vi "Fetch.vi"(8 "error in (no error)":errorcluster, 10 "Message in":refnum<class "FetchMessage.lvclass">, 11 "ExampleClassDScaffold in":refnum<class "ExampleClassDScaffold.lvclass">) -> (0 "error out":errorcluster, 3 "ExampleClassDScaffold out":refnum<class "ExampleClassDScaffold.lvclass">)   [LabVIEW 2012, in "ExampleClassDScaffold.lvclass"]
doc: "The fetch method processes the command 'fetch'.\n\nThe command 'fetch' is used for receiving various forms of data."
uses:
  ExampleClassDScaffold.lvclass
  <vilib>/Distrio/Murmex/FetchMessage/FetchMessage.lvclass
  <vilib>/Distrio/Murmex/Murmex/Murmex.lvclass
  <vilib>/Distrio/Murmex/Murmex/observer_cluster_2.ctl
  <vilib>/Distrio/Murmex/Murmex/observe_mode_enum.ctl
  <vilib>/Distrio/Murmex/Murmex/Queue type enum.ctl
  <vilib>/Distrio/Murmex/ProceedMessage/ProceedMessage.lvclass
  <vilib>/Distrio/Murmex/Message/Message.lvclass
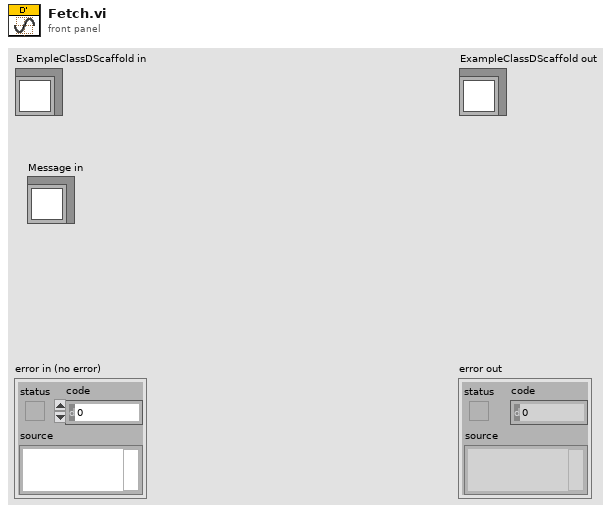
[diagram p1: front panel]
types:
  T1 = typedef "Murmex.lvlib/Murmex.lvclass/Queue type enum.ctl" = enum16{"RabbitMQ", "Network streaming queue"}
  T2 = typedef "Murmex.lvlib/Murmex.lvclass/observe_mode_enum.ctl" = enum16{"all data blocks", "only finished data blocks"}
  T3 = typedef "Murmex.lvlib/Murmex.lvclass/observer_cluster_2.ctl" = cluster{"ID":string, "observe mode":T2, "channels":string, "queue type":T1, "wait until done?":bool}
  T4 = typedef "Murmex.lvlib/FetchMessage.lvclass/Channel data cluster.ctl" = cluster{"channel id":i32, "data UInt8":u8[], "data type":T5, "dimensions":i32[], "physical units":T6[], "waveform dt":dbl, "waveform":T7}
  T5 = typedef "Murmex.lvlib/Murmex.lvclass/data_type_enum.ctl" = enum16{"Float128", "Float64", "Float32", "Int64", "Int32", "Int16", "Int8", "UInt64", "UInt32", "UInt16", "UInt8", "Boolean", "String"}
  T6 = typedef "Murmex.lvlib/Murmex.lvclass/Physical Units.ctl" = cluster{"Base Units":enum16{"radian", "steradian", "second", "meter", "kilogram", "ampere", "kelvin", "mole", "candela"}, "Exponent":i16}
  T7 = typedef "Murmex.lvlib/Murmex.lvclass/waveform_type_enum.ctl" = enum16{"no waveform", "analog", "digital"}
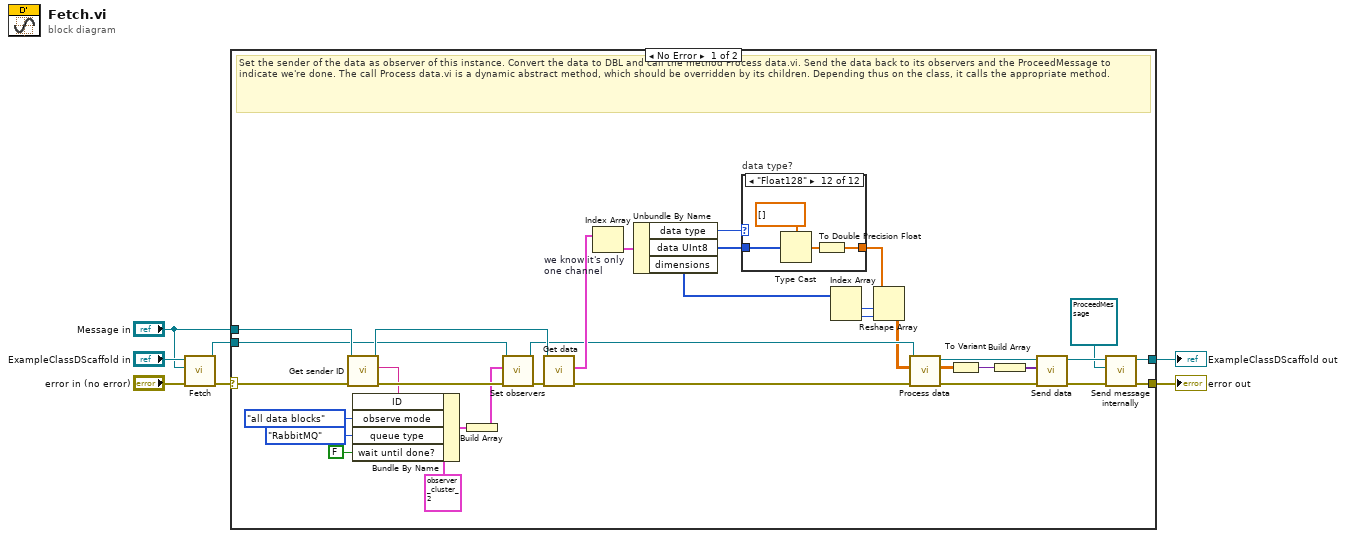
[diagram p0: block diagram]
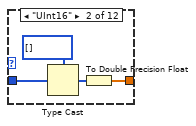
[diagram p3: hidden frame]
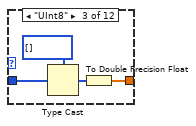
[diagram p4: hidden frame]
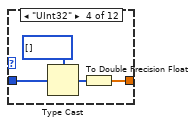
[diagram p5: hidden frame]
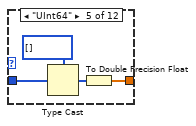
[diagram p6: hidden frame]
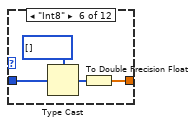
[diagram p7: hidden frame]
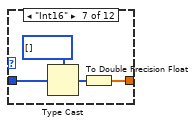
[diagram p8: hidden frame]
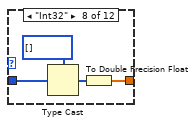
[diagram p9: hidden frame]
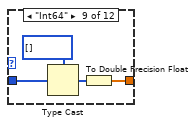
[diagram p10: hidden frame]
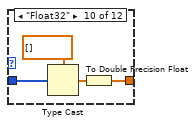
[diagram p11: hidden frame]
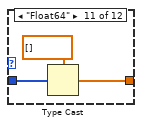
[diagram p12: hidden frame]
diagram:
  n1 = call-parent "Fetch.vi"("error in (no error)"="error in (no error)", "Message in"="Message in", "Murmex in"="ExampleClassDScaffold in") -> ("error out"=w1:errorcluster, "Murmex out"=w3:refnum<class "ExampleClassDScaffold.lvclass">)  [unwired: 7 in]
  n2 = case shown="No Error" w1 {
    selector: w1 -> [w39 w86]
    tunnel: "Message in" -> [w35 _]
    tunnel: [w23 w86] -> w4
    tunnel: w3 -> [w33 w85]
    tunnel: [w21 w85] -> w2
    frame No Error {
      # "Set the sender of the data as observer of this instance. Convert the data to DBL and call the method Process data.vi. Send the data back to its observers and the ProceedMessage to indicate we're done. The call Process data.vi is a dynamic abstract method, which should be overridden by its children. Depending thus on the class, it calls the appropriate method."
      n3 = call <vilib>:"Get sender ID.vi"("error in (no error)"=w39, "Message in"=w35) -> ("error out"=w31:errorcluster, "sender"=w28:string, "Message out"=w34:refnum<class "FetchMessage.lvclass">)  [unwired: 7 in]
      n4 = Bundle By Name(cluster=T3 {"ID"="", "observe mode"=enum."all data blocks", "channels"="", "queue type"=enum."Network streaming queue", "wait until done?"=FALSE} ("observer"), "ID"=w28, "observe mode"=observe_mode_enum."all data blocks", "queue type"=Queue_type_enum."RabbitMQ", "wait until done?"=FALSE) -> (w25:T3)
      n5 = Build Array(w25) -> (w24:T3[])
      n6 = call <vilib>:"Set observers.vi"("error in (no error)"=w31, "observers (component IDs)"=w24, "Murmex in"=w33) -> ("error out"=w30:errorcluster, "Murmex out"=w32:refnum<class "ExampleClassDScaffold.lvclass">)  [unwired: 7 in]
      n7 = call <vilib>:"Get data.vi"("error in (no error)"=w30, "FetchMessage.lvclass"=w34) -> ("error out"=w9:errorcluster, "data (channels)"=w41:T4[])  [unwired: 7 in, 1 out]
      n8 = Index Array "we know it's only\none channel"(array=w41) -> (element=w10:T4)  [unwired: 1 in]
      n9 = Unbundle By Name(w10) -> ("data type"=w18:T5, "data UInt8"=w17:u8[], "dimensions"=w16:i32[])
      n10 = case "data type?" shown="\"Float128\"" w18 {
        tunnel: w17 -> [_ w45 w49 w53 w57 w61 w65 w69 w73 w77 w80 w84]
        tunnel: [_ w42 w46 w50 w54 w58 w62 w66 w70 w74 w78 w81] -> w15
        frame Default {
        }
        frame "UInt16" {
          n11 = Type Cast(type=u16[] [] ("data UInt8"), x=w45) -> (*(type *) &x=w43:u16[])
          n12 = To Double Precision Float(number=w43) -> (double precision float=w42:dbl[])
        }
        frame "UInt8" {
          n13 = Type Cast(type=u8[] [] ("data UInt8"), x=w49) -> (*(type *) &x=w47:u8[])
          n14 = To Double Precision Float(number=w47) -> (double precision float=w46:dbl[])
        }
        frame "UInt32" {
          n15 = Type Cast(type=u32[] [] ("data UInt8"), x=w53) -> (*(type *) &x=w51:u32[])
          n16 = To Double Precision Float(number=w51) -> (double precision float=w50:dbl[])
        }
        frame "UInt64" {
          n17 = Type Cast(type=u64[] [] ("data UInt8"), x=w57) -> (*(type *) &x=w55:u64[])
          n18 = To Double Precision Float(number=w55) -> (double precision float=w54:dbl[])
        }
        frame "Int8" {
          n19 = Type Cast(type=i8[] [] ("data UInt8"), x=w61) -> (*(type *) &x=w59:i8[])
          n20 = To Double Precision Float(number=w59) -> (double precision float=w58:dbl[])
        }
        frame "Int16" {
          n21 = Type Cast(type=i16[] [] ("data UInt8"), x=w65) -> (*(type *) &x=w63:i16[])
          n22 = To Double Precision Float(number=w63) -> (double precision float=w62:dbl[])
        }
        frame "Int32" {
          n23 = Type Cast(type=i32[] [] ("data UInt8"), x=w69) -> (*(type *) &x=w67:i32[])
          n24 = To Double Precision Float(number=w67) -> (double precision float=w66:dbl[])
        }
        frame "Int64" {
          n25 = Type Cast(type=i64[] [] ("data UInt8"), x=w73) -> (*(type *) &x=w71:i64[])
          n26 = To Double Precision Float(number=w71) -> (double precision float=w70:dbl[])
        }
        frame "Float32" {
          n27 = Type Cast(type=sgl[] [] ("data UInt8"), x=w77) -> (*(type *) &x=w75:sgl[])
          n28 = To Double Precision Float(number=w75) -> (double precision float=w74:dbl[])
        }
        frame "Float64" {
          n29 = Type Cast(type=dbl[] [] ("data UInt8"), x=w80) -> (*(type *) &x=w78:dbl[])
        }
        frame "Float128" {
          n30 = Type Cast(type=ext[] [] ("data UInt8"), x=w84) -> (*(type *) &x=w82:ext[])
          n31 = To Double Precision Float(number=w82) -> (double precision float=w81:dbl[])
        }
      }
      n32 = Index Array(array=w16) -> (element #1=w14:i32, element #2=w13:i32)  [unwired: 2 in]
      n33 = Reshape Array(w15, w14, w13) -> (w12:dbl[][])
      n34 = call-dynamic "Process data.vi"("error in (no error)"=w9, "input array"=w12, "ExampleClassDScaffold in"=w32) -> ("error out"=w40:errorcluster, "output array"=w11:dbl[][], "ExampleClassDScaffold out"=w37:refnum<class "ExampleClassDScaffold.lvclass">)  [unwired: 6 in]
      n35 = To Variant(anything=w11) -> (Variant=w36:variant)
      n36 = Build Array(w36) -> (w8:variant[])
      n37 = call <vilib>:"Send data.vi"("error in (no error)"=w40, "data (channels array)"=w8, "Murmex in"=w37) -> ("error out"=w38:errorcluster, "Murmex out"=w22:refnum<class "ExampleClassDScaffold.lvclass">)  [unwired: 7 in]
      n38 = call <vilib>:"Send message internally.vi"("error in (no error)"=w38, "Message"=refnum<class "ProceedMessage.lvclass"> refnum ("Distrio Murmex 1.5:ProceedMessage"), "Murmex in"=w22) -> ("error out"=w23:errorcluster, "Murmex out"=w21:refnum<class "ExampleClassDScaffold.lvclass">)  [unwired: 7 in]
    }
    frame Error {
    }
  }
  "error out" <- w4
  "ExampleClassDScaffold out" <- w2
